vi "Signal analysis.vi"(10 "DBSignal":T1 {"Message_Type" items=["CAN", "CANFD", "J1939"]; "Mux_Type" items=["Normal", "multiplexor", "multiplexed"]; "Is_Motorola" items=["Intel", "Motorola"]; "Value_Type" items=["unsigned int", "signed int", "float", "double"]; "ID" format="%.0x"}, 11 "Value in":string[][](array[string])) -> (3 "Value out":string[][](array[string]))   [LabVIEW 2014]
uses:
  Typedef/DBSignal.ctl
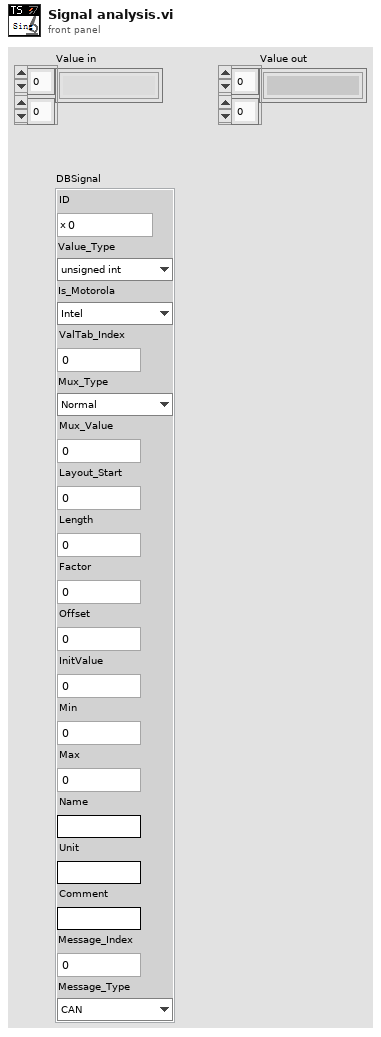
[diagram p1: front panel]
types:
  T1 = typedef "DBSignal.ctl" = cluster{"ID":i32, "Value_Type":i32, "Is_Motorola":i32, "ValTab_Index":i32, "Mux_Type":i32, "Mux_Value":dbl, "Layout_Start":i32, "Length":i32, "Factor":dbl, "Offset":dbl, "InitValue":dbl, "Min":dbl, "Max":dbl, "Name":string, "Unit":string, "Comment":string, "Message_Index":i32, "Message_Type":i32}
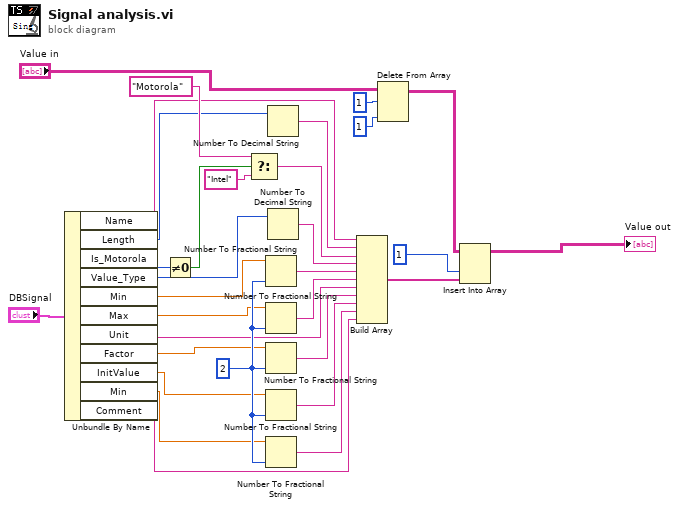
[diagram p0: block diagram]
diagram:
  w24 = i16 2 ("precision (6)")
  n1 = Unbundle By Name("DBSignal") -> ("Name"=w8:string, "Length"=w2:i32, "Is_Motorola"=w27:i32, "Value_Type"=w25:i32, "Min"=w3:dbl, "Max"=w4:dbl, "Unit"=w12:string, "Factor"=w5:dbl, "InitValue"=w6:dbl, "Min"=w7:dbl, "Comment"=w16:string)
  n2 = Not Equal To 0?(x=w27) -> (x != 0?=w28:bool)
  n3 = Select(t="Motorola" ("y"), s=w28, f="Intel" ("y")) -> (s? t:f=w31:string)
  n4 = Number To Fractional String(number=w3, precision (6)=w24) -> (F-format string=w10:string)  [unwired: 2 in]
  n5 = Number To Fractional String(number=w4, precision (6)=w24) -> (F-format string=w11:string)  [unwired: 2 in]
  n6 = Number To Fractional String(number=w5, precision (6)=w24) -> (F-format string=w13:string)  [unwired: 2 in]
  n7 = Number To Fractional String(number=w6, precision (6)=w24) -> (F-format string=w14:string)  [unwired: 2 in]
  n8 = Number To Fractional String(number=w7, precision (6)=w24) -> (F-format string=w15:string)  [unwired: 2 in]
  n9 = Number To Decimal String(number=w2) -> (decimal integer string=w9:string)  [unwired: 1 in]
  n10 = Number To Decimal String(number=w25) -> (decimal integer string=w26:string)  [unwired: 1 in]
  n11 = Build Array(w8, w9, w31, w26, w10, w11, w12, w13, w14, w15, w16) -> (w23:string[])
  n12 = Delete From Array(array="Value in", length=1 ("disabled index (col)"), index (col)=1 ("disabled index (col)")) -> (array with subset deleted=w19:string[][])  [unwired: 1 in, 1 out]
  n13 = Insert Into Array(array=w19, index (col)=1 ("disabled index (col)"), new element=w23) -> (→"Value out":string[][])  [unwired: 1 in]
